vi "Starter Kit FPGA Main.vi"() -> ()   [LabVIEW 2017, in "NI_Robotics_Starter Kit 2.0 FPGA.lvlib"]
doc: "This VI implements the low level control of the motors and sensor for the Starter Kit robot."
uses:
  <vilib>/robotics/Starter Kit/2.0/FPGA Source/NI_Robotics_Starter Kit 2.0 FPGA.lvlib
  <vilib>/Platform/TimedLoop/XDataNode/XDataNode.xnode
  <vilib>/Platform/TimedLoop/XDataNode/nitl_modes.ctl
  <vilib>/Platform/TimedLoop/XDataNode/XDNodeRunTimeDep.lvlib
  <vilib>/Platform/TimedLoop/XDataNode/wakeup.ctl
  <vilib>/Platform/TimedLoop/XDataNode/timing_clust.ctl
  <vilib>/eio/EIONode/EIONode.xnode
  <vilib>/addons/control/pid/fpga.llb/XNode/niFpgaPID.xnode
  <vilib>/robotics/Utilities/Encoder Count Encoding.ctl
  <vilib>/robotics/Utilities/NI_Robotics Utilities.lvlib
  <vilib>/robotics/Utilities/FPGA Utilities/NI_Robotics_FPGA Utilities.lvlib
  <vilib>/robotics/Utilities/FPGA Utilities/Generate Digital Pulse (uSec).vi
  <vilib>/robotics/Starter Kit/FPGA Source/NI_Robotics_Starter Kit FPGA.lvlib
  <vilib>/robotics/Utilities/FPGA Utilities/Count Two Phase Digital Encoder.vi
  <instrlib>/Parallax PING)))/FPGA/NI_Robotics_Parallax PING))) (FPGA).lvlib
  <instrlib>/Sharp IR GP2D12/FPGA/NI_Robotics_Sharp IR GP2D12 (FPGA).lvlib
  <instrlib>/Hitec HS400 Series/FPGA/NI_Robotics_Hitec HS400 Series (FPGA).lvlib
  <vilib>/robotics/Starter Kit/2.0/FPGA Source/Globals.vi
  <vilib>/rvi/eio/common/nirviEmuTemplateMethod_errors.vi
panel:
  in  "FPGA LED":bool
  in  "ModB/AO0":fxp<+/-,20,5> format="%.17g"
  in  "ModB/AO1":fxp<+/-,20,5> format="%.17g"
  in  "ModB/AO2":fxp<+/-,20,5> format="%.17g"
  in  "ModB/AO3":fxp<+/-,20,5> format="%.17g"
  out "ModA/AI0":fxp<+/-,26,5> format="%.23g"
  out "ModA/AI1":fxp<+/-,26,5> format="%.23g"
  out "ModA/AI2":fxp<+/-,26,5> format="%.23g"
  out "ModA/AI3":fxp<+/-,26,5> format="%.23g"
  out "ModA/AI7":fxp<+/-,26,5> format="%.23g"
  out "ModA/AI6":fxp<+/-,26,5> format="%.23g"
  out "ModA/AI5":fxp<+/-,26,5> format="%.23g"
  out "ModA/AI4":fxp<+/-,26,5> format="%.23g"
  out "ModA/AI9":fxp<+/-,26,5> format="%.23g"
  out "ModA/AI8":fxp<+/-,26,5> format="%.23g"
  in  "Port7/DIO0_PWM":T1={"period (us)"=20000, "pulse width (us)"=1500}
  in  "Port7/DIO1_PWM":T1={"period (us)"=20000, "pulse width (us)"=1500}
  in  "Port7/DIO2_PWM":T1={"period (us)"=20000, "pulse width (us)"=1500}
  in  "Port7/DIO3_PWM":T1={"period (us)"=20000, "pulse width (us)"=1500}
  in  "DCmotor_1_direct":bool
  in  "DCmotor_0_direct":bool
  in  "servo_0_direct":bool
  in  "DCmotor_1_PWM":T1={"period (us)"=20000, "pulse width (us)"=1500}
  in  "DCmotor_0_PWM":T1={"period (us)"=20000, "pulse width (us)"=1500}
  in  "servo_0_PWM":T1={"period (us)"=20000, "pulse width (us)"=1500}
  in  "Port3/DIO9":bool
  in  "Port3/DIO9_write":bool
  in  "Port3/DIO8":bool
  in  "Port3/DIO8_write":bool
  in  "Port3/DIO7":bool
  in  "Port3/DIO7_write":bool
  in  "Port3/DIO6":bool
  in  "Port3/DIO6_write":bool
  in  "Port3/DIO5":bool
  in  "Port3/DIO5_write":bool
  in  "Port3/DIO4":bool
  in  "Port3/DIO4_write":bool
  in  "Port3/DIO3":bool
  in  "Port3/DIO3_write":bool
  in  "Port3/DIO2":bool
  in  "Port3/DIO2_write":bool
  in  "Port3/DIO1":bool
  in  "Port3/DIO1_write":bool
  in  "Port3/DIO0":bool
  in  "Port3/DIO0_write":bool
  out "GP2D12_0_voltage":fxp<+/-,26,5> format="%.23g"
  out "GP2D12_0_dist":fxp<+/-,31,13>
  in  "GP2D12_0_calparams":T2={"m"=3.028200149536133, "b"=0.30049991607666016, "k"=0.04309988021850586}
  in  "hs400_0_ccw offset":fxp<+/-,32,4>
  in  "hs400_0_ccw angle":fxp<+/-,32,4>
  out "PING)))_0_timeout":bool
  out "PING)))_0_dist":fxp<+,32,8> format="%.27g"
  out "DCmotor_1_ccw vel":fxp<+/-,32,11>
  out "DCmotor_0_ccw vel":fxp<+/-,32,11>
  in  "DCmotor_1_ccw vel sp":fxp<+/-,32,11>
  in  "DCmotor_0_ccw vel sp":fxp<+/-,32,11>
  in  "stop":bool
  in  "motor PID gains":T3={"proportional gain (Kc)"=0.25, "integral gain (Kc*Ts/Ti)"=0.08984375, "derivative gain (Kc*Td/Ts)"=0.01171875}
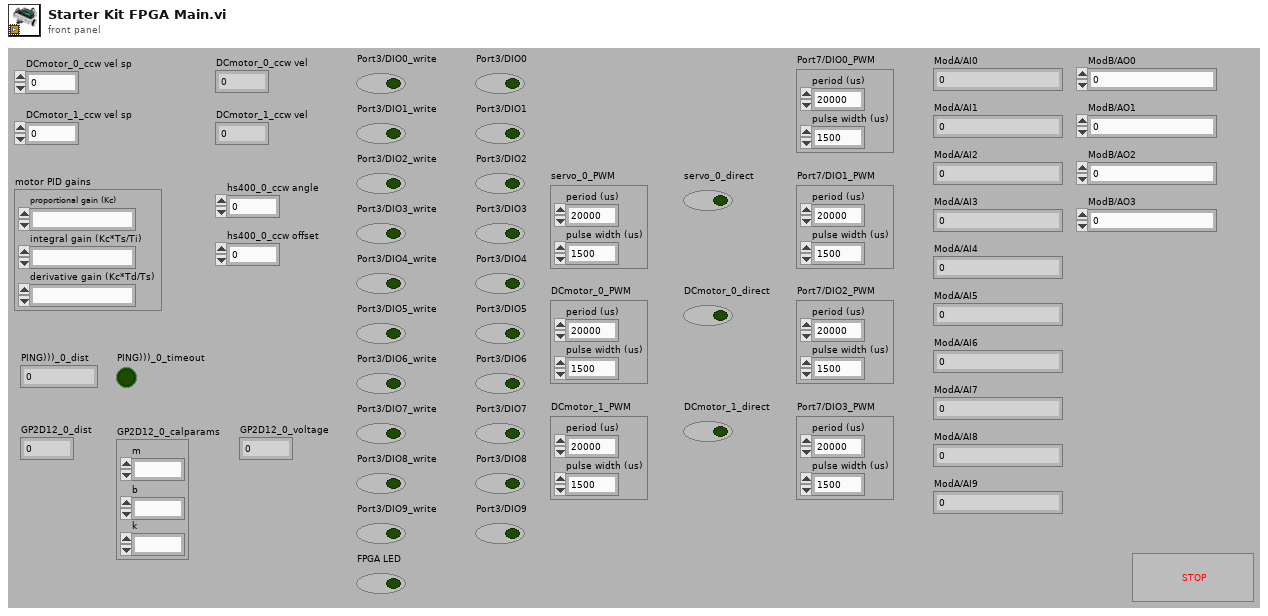
[diagram p1: front panel]
types:
  T1 = cluster{"period (us)":u32, "pulse width (us)":u32}
  T2 = cluster{"m":fxp<+/-,26,5>, "b":fxp<+/-,26,5>, "k":fxp<+/-,26,5>}
  T3 = cluster{"proportional gain (Kc)":fxp<+/-,16,8>, "integral gain (Kc*Ts/Ti)":fxp<+/-,16,8>, "derivative gain (Kc*Td/Ts)":fxp<+/-,16,8>}
  T4 = cluster{"PID gains":cluster{"proportional gain (Kc)":fxp<+/-,16,8>, "integral gain (Kc*Ts/Ti)":fxp<+/-,16,8>, "derivative gain (Kc*Td/Ts)":fxp<+/-,16,8>}, "output range":cluster{"output high":fxp<+/-,16,16>, "output low":fxp<+/-,16,16>}, "setpoint":fxp<+/-,16,16>, "channel index":u16}
  T5 = cluster{"PID gains (x 2^8)":cluster{"proportional gain (Kc)":i16, "integral gain (Kc*Ts/Ti)":i16, "derivative gain (Kc*Td/Ts)":i16}, "output range":cluster{"output high":i16, "output low":i16}, "setpoint":i16, "channel index":u16}
  T6 = typedef "XDNodeRunTimeDep.lvlib/timing_clust.ctl" = cluster{"Expected End [f-1]":u64, "Actual End [f-1]":u64, "Finished Late? [f-1]":bool, "Expected End [i-1]":u64, "Actual End [i-1]":u64, "Finished Late? [i-1]":bool, "Expected Start [i]":u64, "Actual Start [i]":u64, "Expected Start [f]":u64, "Actual Start [f]":u64, "Source Name":string, "Structure Name":string, "Period":i64, "Deadline":i64, "Offset":i64, "Start":i64, "Priority":i32, "Timeout":i32, "Mode":T7, "Wakeup Reason":T8, "Error":errorcluster, "Source Type":string, "Secondary Source Type":string, "Global End Time":u64, "Global Start Time":u64, "Frame Duration":u64, "Iteration Duration":u64, "Assigned CPU":i32, "I/O Scan Engine Mode":u32}
  T7 = typedef "XDNodeRunTimeDep.lvlib/nitl_modes.ctl" = enum32{"No Change", "Process missed periods, maintain original phase", "Discard missed periods, maintain original phase", "Process missed periods, ignore original phase", "Discard missed periods, ignore original phase"}
  T8 = typedef "XDNodeRunTimeDep.lvlib/wakeup.ctl" = enum32{"Normal", "Aborted", "Asynchronous wakeup", "Timing source error", "Timed loop error", "Timeout"}
  T9 = typedef "NI_Robotics Utilities.lvlib/Encoder Count Encoding.ctl" = enum16{"X1", "X2", "X4"}
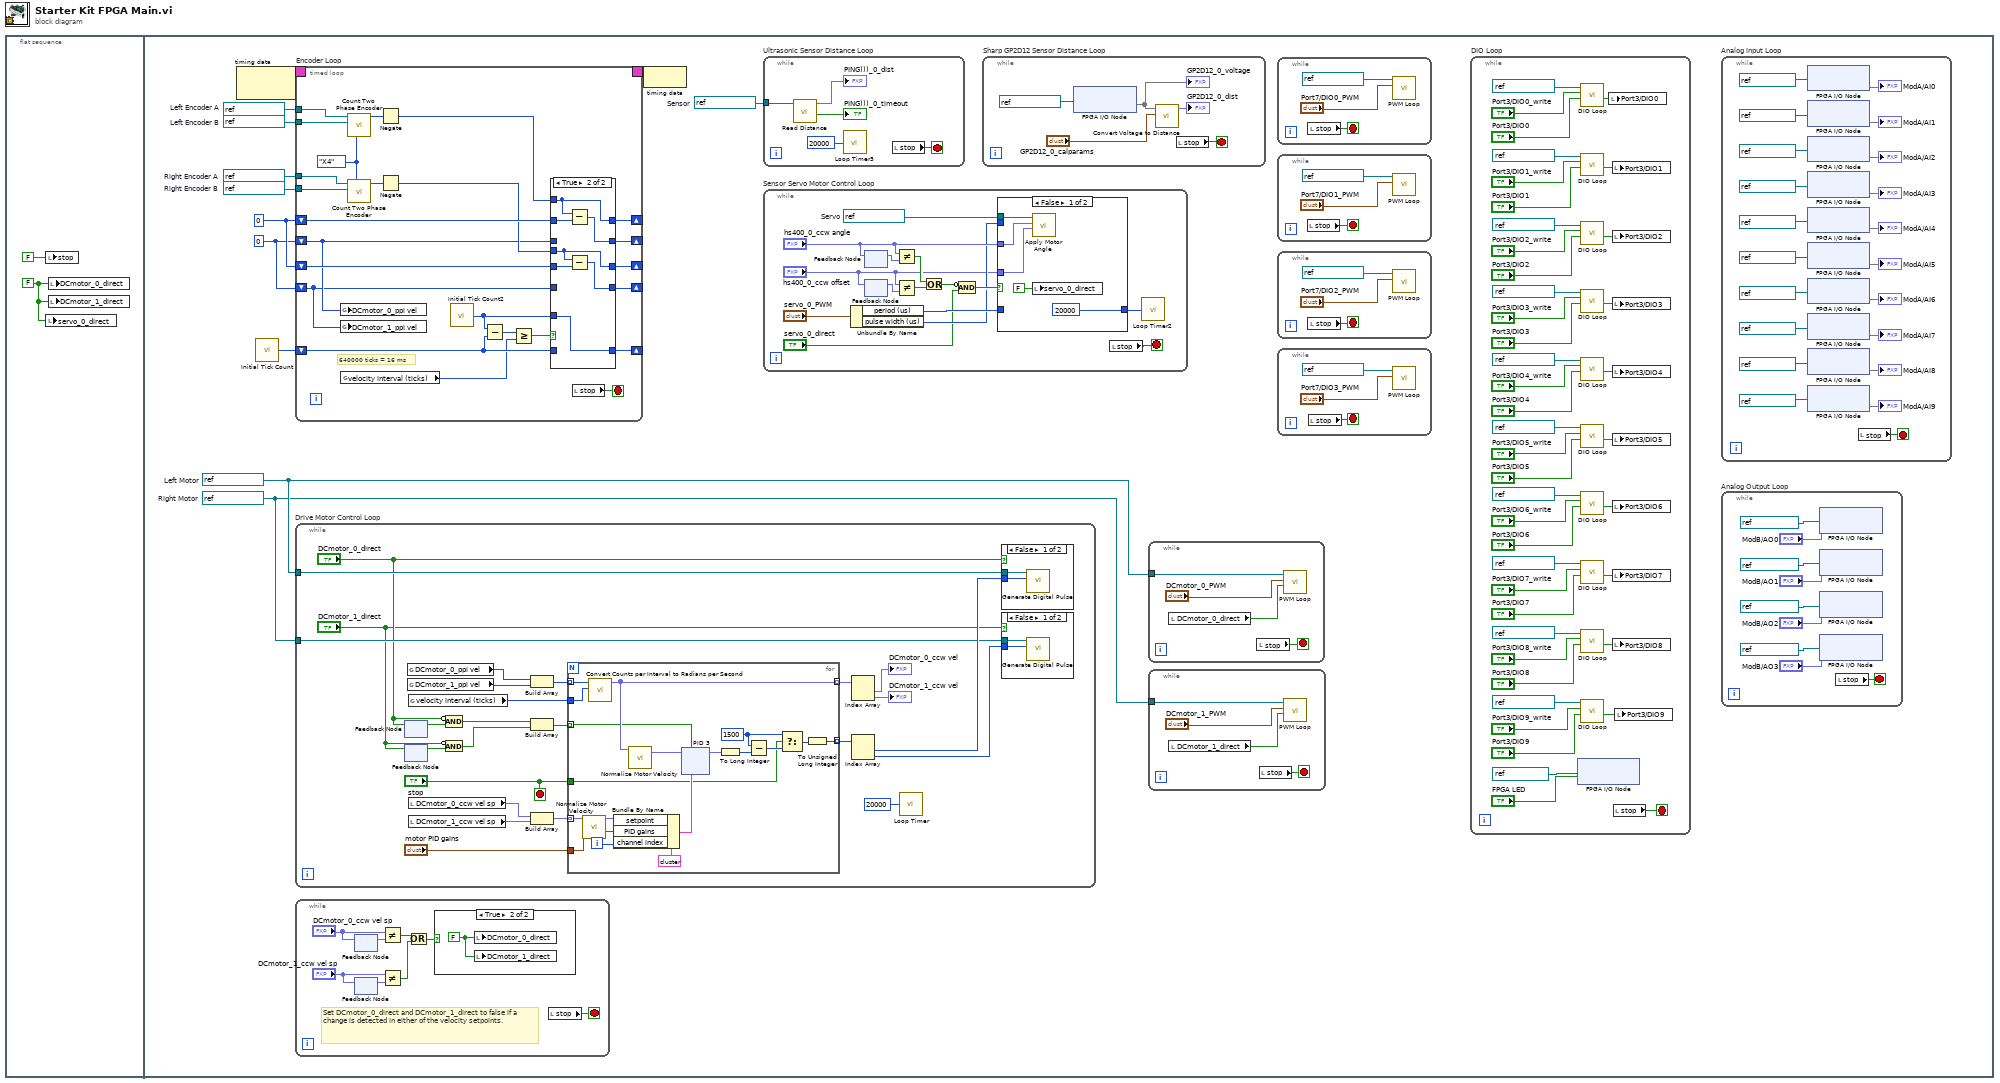
[diagram p0: block diagram]
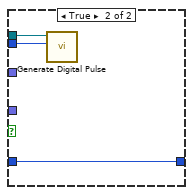
[diagram p5: hidden frame]
diagram:
  n1 = flat-sequence {
    frame #0 {
      w1 = FALSE ("DCmotor_0_direct")
      n2 = local write "stop"(FALSE ("stop")) -> ()
      n3 = local write "servo_0_direct"(w1) -> ()
      n4 = local write "DCmotor_0_direct"(w1) -> ()
      n5 = local write "DCmotor_1_direct"(w1) -> ()
    }
    frame #1 {
      w3 = refnum<k21> "Port0/DIO5"  # Right Motor
      w4 = refnum<k21> "Port0/DIO4"  # Left Motor
      w5 = refnum<k21> "Port0/DIO3"  # Right Encoder B
      w6 = refnum<k21> "Port0/DIO2"  # Right Encoder A
      w7 = refnum<k21> "Port0/DIO1"  # Left Encoder B
      w8 = refnum<k21> "Port0/DIO0"  # Left Encoder A
      w9 = refnum<k21> "Port0/DIO6"  # Sensor
      w10 = 0
      w11 = 0 ("Reset Position Value")
      n6 = node-c288() -> (w14:T6)  [unwired: 1 in]
      n7 = call "Initial Tick Count"() -> ("Tick Count(Ticks)"=w12:u32)
      n8 = while "Drive Motor Control Loop" {
        tunnel: w4 -> [w139]
        tunnel: w3 -> [w135]
        stop <- "stop" stop-if-true
        n9 = feedback #1() -> (w127:bool)  [unwired: 1 in]
        n10 = feedback-in #1("DCmotor_0_direct") -> ()
        n11 = feedback #2() -> (w128:bool)  [unwired: 1 in]
        n12 = feedback-in #2("DCmotor_1_direct") -> ()
        n13 = global read "Globals.vi" "DCmotor_0_ppi vel"() -> (w132:i32)
        n14 = global read "Globals.vi" "DCmotor_1_ppi vel"() -> (w131:i32)
        n15 = global read "Globals.vi" "velocity interval (ticks)"() -> (w130:u32)
        n16 = local read "DCmotor_0_ccw vel sp"() -> (w134:fxp<+/-,32,11>)
        n17 = local read "DCmotor_1_ccw vel sp"() -> (w133:fxp<+/-,32,11>)
        n18 = Compound Arithmetic op=AND(invert "DCmotor_0_direct", w127) -> (w124:bool)
        n19 = Compound Arithmetic op=AND(invert "DCmotor_1_direct", w128) -> (w123:bool)
        n20 = Build Array(w132, w131) -> (w144:i32[])
        n21 = Build Array(w124, w123) -> (w122:bool[])
        n22 = Build Array(w134, w133) -> (w142:fxp<+/-,32,11>[])
        n23 = for {
          tunnel: "motor PID gains" -> [w165]
          tunnel: w144 -> [w164] mode=indexing
          tunnel: w130 -> [w163]
          tunnel: [w162] -> w143 mode=indexing
          tunnel: w142 -> [w159] mode=indexing
          tunnel: "stop" -> [w152]
          tunnel: [w153] -> w141 mode=indexing
          tunnel: w122 -> [w151] mode=indexing
          i -> [w166]
          w156 = 1500 ("y")
          n24 = call <vilib>:"Normalize Motor Velocity.vi"("velocity (rad/s)"=w159) -> ("normalized velocity"=w160:fxp<+/-,16,16>)  [unwired: 10 in]
          n25 = call <vilib>:"Convert Counts per Interval to Radians per Second.vi"("interval (ticks)"=w163, "velocity (pulses/interval)"=w164) -> ("velocity (rad/s)"=w162:fxp<+/-,32,11>)  [unwired: 9 in]
          n26 = Bundle By Name(cluster=T4 {"PID gains"={"proportional gain (Kc)"=0.00390625, "integral gain (Kc*Ts/Ti)"=0.00390625, "derivative gain (Kc*Td/Ts)"=0.00390625}, "output range"={"output high"=500.0, "output low"=-500.0}, "setpoint"=0.0, "channel index"=0} ("configuration"), "setpoint"=w160, "PID gains"=w165, "channel index"=w166) -> (w167:T4)
          n27 = call <vilib>:"Normalize Motor Velocity.vi"("velocity (rad/s)"=w162) -> ("normalized velocity"=w161:fxp<+/-,16,16>)  [unwired: 10 in]
          n28 = xnode ("PID 3")("process variable"=w161, "reset?"=w151, "configuration"=w167) -> ("output"=w154:fxp<+/-,16,16>)  [unwired: 1 out]
          n29 = To Long Integer(number=w154) -> (32bit integer=w155:i32)
          n30 = Subtract(x=w156, y=w155) -> (x-y=w157:i32)
          n31 = Select(t=w156, s=w152, f=w157) -> (s? t:f=w158:i32)
          n32 = To Unsigned Long Integer(number=w158) -> (unsigned 32bit integer=w153:u32)
        }
        n33 = Index Array(array=w143) -> (element #1=→"DCmotor_0_ccw vel":fxp<+/-,32,11>, element #2=→"DCmotor_1_ccw vel":fxp<+/-,32,11>)  [unwired: 2 in]
        n34 = Index Array(array=w141) -> (element #1=w140:u32, element #2=w136:u32)  [unwired: 2 in]
        n35 = call "Loop Timer"("Count(uSec)"=u32 20000) -> ()  [unwired: 1 out]
        n36 = case shown="False" "DCmotor_0_direct" {
          tunnel: w140 -> [w150 _]
          tunnel: w139 -> [w149 _]
          frame False {
            n37 = call-poly <vilib>:"Generate Digital Pulse.vi"("pulse width (uSec)"=w150, "FPGA digital output"=w149) -> ()  [unwired: 10 in]
          }
          frame True {
          }
        }
        n38 = case shown="False" "DCmotor_1_direct" {
          tunnel: w136 -> [w148 _]
          tunnel: w135 -> [w147 _]
          frame False {
            n39 = call-poly <vilib>:"Generate Digital Pulse.vi"("pulse width (uSec)"=w148, "FPGA digital output"=w147) -> ()  [unwired: 10 in]
          }
          frame True {
          }
        }
      }
      n40 = while {
        stop <- w20 stop-if-true
        # "Set DCmotor_0_direct and DCmotor_1_direct to false if a change is detected in either of the velocity setpoints."
        n41 = feedback-in #3("DCmotor_0_ccw vel sp") -> ()
        n42 = feedback #3() -> (w22:fxp<+/-,32,11>)  [unwired: 1 in]
        n43 = feedback #4() -> (w18:fxp<+/-,32,11>)  [unwired: 1 in]
        n44 = feedback-in #4("DCmotor_1_ccw vel sp") -> ()
        n45 = Not Equal?(x="DCmotor_0_ccw vel sp", y=w22) -> (x != y?=w16:bool)
        n46 = Not Equal?(x="DCmotor_1_ccw vel sp", y=w18) -> (x != y?=w17:bool)
        n47 = Or(x=w16, y=w17) -> (x .or. y?=w15:bool)
        n48 = case shown="True" w15 {
          frame False {
          }
          frame True {
            w23 = FALSE ("DCmotor_0_direct")
            n49 = local write "DCmotor_0_direct"(w23) -> ()
            n50 = local write "DCmotor_1_direct"(w23) -> ()
          }
        }
        n51 = local read "stop"() -> (w20:bool)
      }
      n52 = timed-loop "Encoder Loop" {
        timing: w14 -> [_]
        timing-out: [_] -> w13
        shift-right: [w240] -> _
        shift-left: w12 -> [w245]
        shift-right: [w241] -> _
        shift-left: w11 -> [w243]
        shift-right: [w242] -> _
        shift-left: w10 -> [w227]
        shift-right: [w238] -> _
        shift-left: w11 -> [w239]
        shift-right: [w237] -> _
        shift-left: w10 -> [w226]
        tunnel: w8 -> [w234]
        tunnel: w7 -> [w233]
        tunnel: w6 -> [w231]
        tunnel: w5 -> [w230]
        stop <- w224 stop-if-true
        w228 = Encoder_Count_Encoding."X4" ("count multiplier (X1)")
        # "640000 ticks = 16 ms"
        n53 = global write "Globals.vi" "DCmotor_0_ppi vel"(w227) -> ()
        n54 = global write "Globals.vi" "DCmotor_1_ppi vel"(w226) -> ()
        n55 = global read "Globals.vi" "velocity interval (ticks)"() -> (w225:u32)
        n56 = call-poly <vilib>:"Count Two Phase Encoder.vi"("count encoding (X1)"=w228, "phase B FPGA digital input"=w233, "phase A FPGA digital input"=w234) -> ("new count"=w232:i32)  [unwired: 7 in, 1 out]
        n57 = call-poly <vilib>:"Count Two Phase Encoder.vi"("count encoding (X1)"=w228, "phase B FPGA digital input"=w230, "phase A FPGA digital input"=w231) -> ("new count"=w229:i32)  [unwired: 7 in, 1 out]
        n58 = Negate(x=w232) -> (-x=w236:i32)
        n59 = Negate(x=w229) -> (-x=w235:i32)
        n60 = call "Initial Tick Count2"() -> ("Tick Count(Ticks)"=w244:u32)
        n61 = Subtract(x=w244, y=w245) -> (x-y=w247:u32)
        n62 = Greater Or Equal?(x=w247, y=w225) -> (x >= y?=w246:bool)
        n63 = case shown="True" w246 {
          tunnel: w244 -> [_ w258]
          tunnel: w245 -> [w252 _]
          tunnel: [w252 w258] -> w240
          tunnel: w243 -> [w251 w259]
          tunnel: [w251 w257] -> w241
          tunnel: w236 -> [_ w257]
          tunnel: [w250 w256] -> w242
          tunnel: w227 -> [w250 _]
          tunnel: w239 -> [w249 w255]
          tunnel: w226 -> [w248 _]
          tunnel: [w249 w254] -> w238
          tunnel: [w248 w253] -> w237
          tunnel: w235 -> [_ w254]
          frame False {
          }
          frame True {
            n64 = Subtract(x=w257, y=w259) -> (x-y=w256:i32)
            n65 = Subtract(x=w254, y=w255) -> (x-y=w253:i32)
          }
        }
        n66 = local read "stop"() -> (w224:bool)
      }
      n67 = node-c288(w13) -> ()
      n68 = while "Ultrasonic Sensor Distance Loop" {
        tunnel: w9 -> [w222]
        stop <- w219 stop-if-true
        n69 = call <instrlib>:"Read Distance.vi"("trigger/echo line"=w222) -> ("timed out?"=→"PING)))_0_timeout":bool, "distance (m)"=→"PING)))_0_dist":fxp<+,32,8>)  [unwired: 9 in]
        n70 = call "Loop Timer3"("Count(uSec)"=u32 20000 ("sensor period (15000 us)")) -> ()  [unwired: 1 out]
        n71 = local read "stop"() -> (w219:bool)
      }
      n72 = while "Sensor Servo Motor Control Loop" {
        stop <- w196 stop-if-true
        w209 = refnum<k21> "Port0/DIO7"  # Servo
        n73 = Unbundle By Name("servo_0_PWM") -> ("period (us)"=w207:u32, "pulse width (us)"=w199:u32)
        n74 = feedback #5() -> (w205:fxp<+/-,32,4>)  [unwired: 1 in]
        n75 = feedback-in #5("hs400_0_ccw angle") -> ()
        n76 = feedback #6() -> (w204:fxp<+/-,32,4>)  [unwired: 1 in]
        n77 = feedback-in #6("hs400_0_ccw offset") -> ()
        n78 = Not Equal?(x="hs400_0_ccw angle", y=w205) -> (x != y?=w202:bool)
        n79 = Not Equal?(x="hs400_0_ccw offset", y=w204) -> (x != y?=w203:bool)
        n80 = Or(x=w202, y=w203) -> (x .or. y?=w201:bool)
        n81 = Compound Arithmetic op=AND(invert w201, "servo_0_direct") -> (w200:bool)
        n82 = case shown="False" w200 {
          tunnel: w199 -> [_ w218]
          tunnel: w209 -> [w213 w217]
          tunnel: "hs400_0_ccw angle" -> [w212 _]
          tunnel: "hs400_0_ccw offset" -> [w211 _]
          tunnel: [u32 20000 ("Count(uSec)") w216] -> w208
          tunnel: w207 -> [_ w216]
          frame False {
            n83 = call <instrlib>:"Apply Motor Angle.vi"("ccw angle offset (rad)"=w211, "ccw angle (rad)"=w212, "digital output line"=w213) -> ()  [unwired: 9 in]
            n84 = local write "servo_0_direct"(FALSE ("servo_0_direct")) -> ()
          }
          frame True {
            n85 = call-poly <vilib>:"Generate Digital Pulse.vi"("pulse width (uSec)"=w218, "FPGA digital output"=w217) -> ()  [unwired: 10 in]
          }
        }
        n86 = local read "stop"() -> (w196:bool)
        n87 = call "Loop Timer2"("Count(uSec)"=w208) -> ()  [unwired: 1 out]
      }
      n88 = while "Sharp GP2D12 Sensor Distance Loop" {
        stop <- w105 stop-if-true
        n89 = xnode "FPGA I/O Node"("FPGA I/O In"=refnum<k21> "ModA/AI10") -> ("I/O Item"=w106)  [unwired: 1 out]
        "GP2D12_0_voltage" <- w106
        n90 = call <instrlib>:"Convert Voltage to Distance.vi"("calibration parameters"="GP2D12_0_calparams", "voltage"=w106) -> ("distance (m)"=→"GP2D12_0_dist":fxp<+/-,31,13>)  [unwired: 9 in]
        n91 = local read "stop"() -> (w105:bool)
      }
      n92 = while {
        tunnel: w4 -> [w103]
        stop <- w101 stop-if-true
        n93 = local read "DCmotor_0_direct"() -> (w102:bool)
        n94 = local read "stop"() -> (w101:bool)
        n95 = call <vilib>:"PWM Loop.vi"("generate pulse (T)"=w102, "PWM"="DCmotor_0_PWM", "FPGA I/O"=w103) -> ()  [unwired: 9 in]
      }
      n96 = while {
        tunnel: w3 -> [w100]
        stop <- w97 stop-if-true
        n97 = local read "DCmotor_1_direct"() -> (w98:bool)
        n98 = local read "stop"() -> (w97:bool)
        n99 = call <vilib>:"PWM Loop.vi"("generate pulse (T)"=w98, "PWM"="DCmotor_1_PWM", "FPGA I/O"=w100) -> ()  [unwired: 9 in]
      }
      n100 = while {
        stop <- w119 stop-if-true
        n101 = local read "stop"() -> (w119:bool)
        n102 = call <vilib>:"PWM Loop.vi"("PWM"="Port7/DIO0_PWM", "FPGA I/O"=refnum<k21> "Port7/DIO0" ("FPGA I/O In")) -> ()  [unwired: 10 in]
      }
      n103 = while {
        stop <- w116 stop-if-true
        n104 = local read "stop"() -> (w116:bool)
        n105 = call <vilib>:"PWM Loop.vi"("PWM"="Port7/DIO1_PWM", "FPGA I/O"=refnum<k21> "Port7/DIO1" ("FPGA I/O In")) -> ()  [unwired: 10 in]
      }
      n106 = while {
        stop <- w113 stop-if-true
        n107 = local read "stop"() -> (w113:bool)
        n108 = call <vilib>:"PWM Loop.vi"("PWM"="Port7/DIO2_PWM", "FPGA I/O"=refnum<k21> "Port7/DIO2" ("FPGA I/O In")) -> ()  [unwired: 10 in]
      }
      n109 = while {
        stop <- w110 stop-if-true
        n110 = local read "stop"() -> (w110:bool)
        n111 = call <vilib>:"PWM Loop.vi"("PWM"="Port7/DIO3_PWM", "FPGA I/O"=refnum<k21> "Port7/DIO3" ("FPGA I/O In")) -> ()  [unwired: 10 in]
      }
      n112 = while "DIO Loop" {
        stop <- w54 stop-if-true
        n113 = xnode "FPGA I/O Node"("I/O Item"="FPGA LED", "FPGA I/O In"=refnum<k21> "FPGA LED" ("LED")) -> ()  [unwired: 1 out]
        n114 = call <vilib>:"DIO Loop.vi"("DIO value in"="Port3/DIO0", "enable output"="Port3/DIO0_write", "DIO line"=refnum<k21> "Port3/DIO0" ("FPGA I/O")) -> ("DIO value out"=w93:bool)  [unwired: 8 in]
        n115 = call <vilib>:"DIO Loop.vi"("DIO value in"="Port3/DIO1", "enable output"="Port3/DIO1_write", "DIO line"=refnum<k21> "Port3/DIO1" ("FPGA I/O")) -> ("DIO value out"=w92:bool)  [unwired: 8 in]
        n116 = call <vilib>:"DIO Loop.vi"("DIO value in"="Port3/DIO2", "enable output"="Port3/DIO2_write", "DIO line"=refnum<k21> "Port3/DIO2" ("FPGA I/O")) -> ("DIO value out"=w85:bool)  [unwired: 8 in]
        n117 = call <vilib>:"DIO Loop.vi"("DIO value in"="Port3/DIO3", "enable output"="Port3/DIO3_write", "DIO line"=refnum<k21> "Port3/DIO3" ("FPGA I/O")) -> ("DIO value out"=w84:bool)  [unwired: 8 in]
        n118 = call <vilib>:"DIO Loop.vi"("DIO value in"="Port3/DIO4", "enable output"="Port3/DIO4_write", "DIO line"=refnum<k21> "Port3/DIO4" ("FPGA I/O")) -> ("DIO value out"=w77:bool)  [unwired: 8 in]
        n119 = call <vilib>:"DIO Loop.vi"("DIO value in"="Port3/DIO5", "enable output"="Port3/DIO5_write", "DIO line"=refnum<k21> "Port3/DIO5" ("FPGA I/O")) -> ("DIO value out"=w76:bool)  [unwired: 8 in]
        n120 = call <vilib>:"DIO Loop.vi"("DIO value in"="Port3/DIO6", "enable output"="Port3/DIO6_write", "DIO line"=refnum<k21> "Port3/DIO6" ("FPGA I/O")) -> ("DIO value out"=w69:bool)  [unwired: 8 in]
        n121 = call <vilib>:"DIO Loop.vi"("DIO value in"="Port3/DIO7", "enable output"="Port3/DIO7_write", "DIO line"=refnum<k21> "Port3/DIO7" ("FPGA I/O")) -> ("DIO value out"=w68:bool)  [unwired: 8 in]
        n122 = call <vilib>:"DIO Loop.vi"("DIO value in"="Port3/DIO8", "enable output"="Port3/DIO8_write", "DIO line"=refnum<k21> "Port3/DIO8" ("FPGA I/O")) -> ("DIO value out"=w61:bool)  [unwired: 8 in]
        n123 = call <vilib>:"DIO Loop.vi"("DIO value in"="Port3/DIO9", "enable output"="Port3/DIO9_write", "DIO line"=refnum<k21> "Port3/DIO9" ("FPGA I/O")) -> ("DIO value out"=w60:bool)  [unwired: 8 in]
        n124 = local write "Port3/DIO0"(w93) -> ()
        n125 = local write "Port3/DIO1"(w92) -> ()
        n126 = local write "Port3/DIO2"(w85) -> ()
        n127 = local write "Port3/DIO3"(w84) -> ()
        n128 = local write "Port3/DIO4"(w77) -> ()
        n129 = local write "Port3/DIO5"(w76) -> ()
        n130 = local write "Port3/DIO6"(w69) -> ()
        n131 = local write "Port3/DIO7"(w68) -> ()
        n132 = local write "Port3/DIO8"(w61) -> ()
        n133 = local read "stop"() -> (w54:bool)
        n134 = local write "Port3/DIO9"(w60) -> ()
      }
      n135 = while "Analog Input Loop" {
        stop <- w33 stop-if-true
        n136 = xnode "FPGA I/O Node"("FPGA I/O In"=refnum<k21> "ModA/AI0") -> ("I/O Item"=→"ModA/AI0")  [unwired: 1 out]
        n137 = xnode "FPGA I/O Node"("FPGA I/O In"=refnum<k21> "ModA/AI1") -> ("I/O Item"=→"ModA/AI1")  [unwired: 1 out]
        n138 = xnode "FPGA I/O Node"("FPGA I/O In"=refnum<k21> "ModA/AI2") -> ("I/O Item"=→"ModA/AI2")  [unwired: 1 out]
        n139 = xnode "FPGA I/O Node"("FPGA I/O In"=refnum<k21> "ModA/AI3") -> ("I/O Item"=→"ModA/AI3")  [unwired: 1 out]
        n140 = xnode "FPGA I/O Node"("FPGA I/O In"=refnum<k21> "ModA/AI4") -> ("I/O Item"=→"ModA/AI4")  [unwired: 1 out]
        n141 = xnode "FPGA I/O Node"("FPGA I/O In"=refnum<k21> "ModA/AI5") -> ("I/O Item"=→"ModA/AI5")  [unwired: 1 out]
        n142 = xnode "FPGA I/O Node"("FPGA I/O In"=refnum<k21> "ModA/AI6") -> ("I/O Item"=→"ModA/AI6")  [unwired: 1 out]
        n143 = xnode "FPGA I/O Node"("FPGA I/O In"=refnum<k21> "ModA/AI7") -> ("I/O Item"=→"ModA/AI7")  [unwired: 1 out]
        n144 = xnode "FPGA I/O Node"("FPGA I/O In"=refnum<k21> "ModA/AI8") -> ("I/O Item"=→"ModA/AI8")  [unwired: 1 out]
        n145 = xnode "FPGA I/O Node"("FPGA I/O In"=refnum<k21> "ModA/AI9") -> ("I/O Item"=→"ModA/AI9")  [unwired: 1 out]
        n146 = local read "stop"() -> (w33:bool)
      }
      n147 = while "Analog Output Loop" {
        stop <- w24 stop-if-true
        n148 = xnode "FPGA I/O Node"("I/O Item"="ModB/AO0", "FPGA I/O In"=refnum<k21> "ModB/AO0") -> ()  [unwired: 1 out]
        n149 = xnode "FPGA I/O Node"("I/O Item"="ModB/AO1", "FPGA I/O In"=refnum<k21> "ModB/AO1") -> ()  [unwired: 1 out]
        n150 = xnode "FPGA I/O Node"("I/O Item"="ModB/AO2", "FPGA I/O In"=refnum<k21> "ModB/AO2") -> ()  [unwired: 1 out]
        n151 = xnode "FPGA I/O Node"("I/O Item"="ModB/AO3", "FPGA I/O In"=refnum<k21> "ModB/AO3") -> ()  [unwired: 1 out]
        n152 = local read "stop"() -> (w24:bool)
      }
    }
  }
